vi "Update Weights.vi"(5 "Beta":fxp<+/-,32,24> format="%.16g", 7 "Error In":fxp<+/-,32,24> format="%.31g", 9 "Taps":refnum<k21>, 11 "Weights":refnum<k21>) -> (1 "Taps Out":refnum<k21>, 3 "Weights Out":refnum<k21>)   [LabVIEW 2013]
uses:
  <vilib>/rvi/Emulation/niFpgaSctlEmulationGetInTimedLoop.vi
  <vilib>/rvi/Emulation/niFpgaEmulationReportErrorSimple.vi
  <vilib>/rvi/Emulation/niFpgaGetClockAttributes.vi
  <vilib>/rvi/DataTransferAndStorage/Container/Common/niFpgaContainerExecOnDevCompGetState.vi
  <vilib>/rvi/Memory/Memory_Emulation/nirvimemoryFastEmulationFpgaImpl.vi
  <instcachedir>/0/nirvimemoryFastEmulationFpgaImpl_5FBAB50466BC4C939F684F8805638BFC.lvgen/nirvimemoryFastEmulationFpgaImpl_5FBAB50466BC4C939F684F8805638BFC_007.vi
  <vilib>/rvi/DataTransferAndStorage/Container/Common/niFpgaContainerGetUniqueNameForEmu.vi
  <vilib>/rvi/Memory/Memory_Emulation/niFpgaMemoryEmulationCacheClearOnFirstRun.vi
  <vilib>/rvi/Memory/Memory_Emulation/nirvimemoryEmulationManagerCache_MakeExclusive.vi
  <vilib>/rvi/Memory/Memory_Emulation/niFpgaMemoryEmulationValidateCache.vi
  <vilib>/rvi/Memory/Memory_Emulation/nirvimemoryEmulationManagerCache_ReleaseExclusive.vi
  <vilib>/rvi/Memory/Memory_Emulation/nirvimemoryEmulationManagerCache_InsertValue.vi
  <vilib>/Utility/error.llb/Clear Errors.vi
  <vilib>/rvi/Memory/Memory_Emulation/nirvimemoryEmulationManagerCache_GetValue.vi
  <vilib>/rvi/Memory/Memory_Emulation/nirvimemoryEmulationManagerCache_SetValue.vi
  <vilib>/rvi/Emulation/niFpgaSctlEmulationResourceMgr.vi
  <vilib>/rvi/Emulation/niFpgaCriticalErrorInLSC.vi
  <vilib>/rvi/DataTransferAndStorage/Container/XNode/niFpgaContainer.xnode
  <vilib>/rvi/Memory/Memory_Emulation/niFpgaMemoryEmulationRefIn.vi
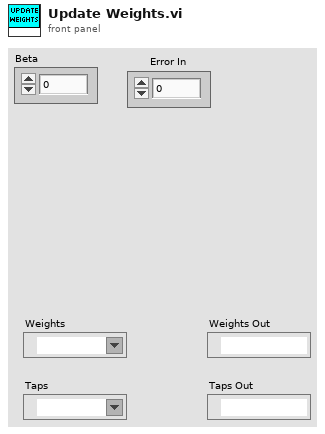
[diagram p1: front panel]
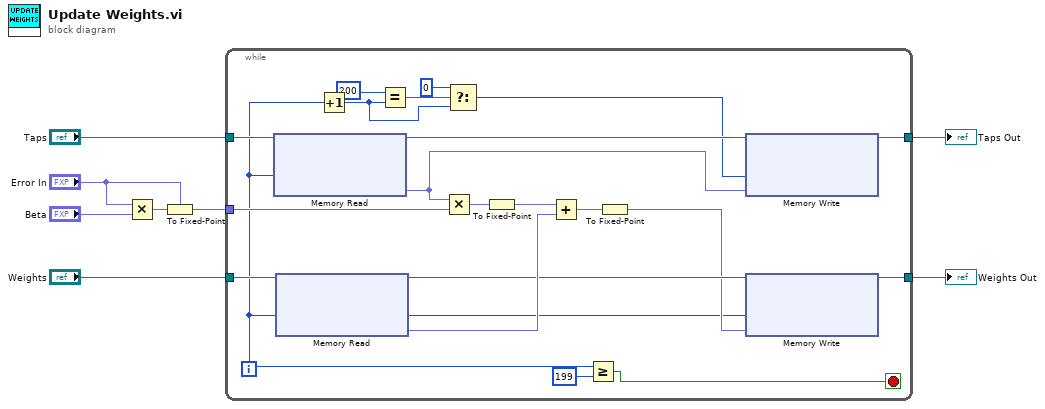
[diagram p0: block diagram]
diagram:
  n1 = Multiply(x="Error In", y="Beta") -> (x*y=w8:fxp<+/-,64,48>)
  n2 = To Fixed-Point(fixed-point type="Error In", number=w8) -> (fixed-point=w4:fxp<+/-,32,24>)
  n3 = while {
    tunnel: "Taps" -> [w29]
    tunnel: w4 -> [w28]
    tunnel: "Weights" -> [w27]
    tunnel: [w22] -> w2
    tunnel: [w15] -> w1
    i -> [w11]
    stop <- w9 stop-if-true
    n4 = xnode ("Memory Read")("Address"=w11, "Memory In"=w29) -> ("Data"=w16:fxp<+/-,32,24>, "Memory Out"=w18:refnum<k21>)
    n5 = xnode ("Memory Read")("Address"=w11, "Memory In"=w27) -> ("Data"=w25:fxp<+/-,32,24>, "Memory Out"=w24:refnum<k21>)
    n6 = Increment(x=w11) -> (x+1=w20:i32)
    n7 = Equal?(x=200, y=w20) -> (x = y?=w21:bool)
    n8 = Multiply(x=w16, y=w28) -> (x*y=w26:fxp<+/-,64,48>)
    n9 = Select(t=0, s=w21, f=w20) -> (s? t:f=w17:i32)
    n10 = To Fixed-Point(number=w26) -> (fixed-point=w14:fxp<+/-,32,24>)  [unwired: 1 in]
    n11 = Add(x=w14, y=w25) -> (x+y=w23:fxp<+/-,33,25>)
    n12 = Greater Or Equal?(x=w11, y=199) -> (x >= y?=w9:bool)
    n13 = To Fixed-Point(number=w23) -> (fixed-point=w13:fxp<+/-,32,24>)  [unwired: 1 in]
    n14 = xnode ("Memory Write")("Address"=w17, "Data"=w16, "Memory In"=w18) -> ("Memory Out"=w15:refnum<k21>)
    n15 = xnode ("Memory Write")("Address"=w11, "Data"=w13, "Memory In"=w24) -> ("Memory Out"=w22:refnum<k21>)
  }
  "Taps Out" <- w1
  "Weights Out" <- w2
